vi "Scale Controls Helper.vi"(5 "rules":string, 6 "Action (Initialize)":enum16{"Initialize", "Resize", "Resize?"}(ring), 8 "error in (no error)":errorcluster, 9 "Force align? (False)":bool, 11 "vi reference":refnum<vi>) -> (0 "error out":errorcluster)   [LabVIEW 2020]
doc: "Helper VI to implement Scale Controls.vi - top level function to be called.\n\n1) Call once at GUI VI startup to initialize with action Initialize.\n2) Then call with action Resize in pane resize event to record new pane size.\n3) Then call in timeout loop with action Resize? to check if there is resize event pending and execute it. In this case the scaling rules string for Scale Controls.vi must be provided!\n\nInput parameters are static VI ref to GUI panel to be scaled in 3) the scaling rules string.\nUse 'Force align' option to force execution of scaler even if pane size not changed."
uses:
  <vilib>/Utility/miscctls.llb/LVRectTypeDef.ctl
panel:
  in  "vi list":cluster{"vi ref":refnum<vi>, "bounds":T1}[](array[cluster])
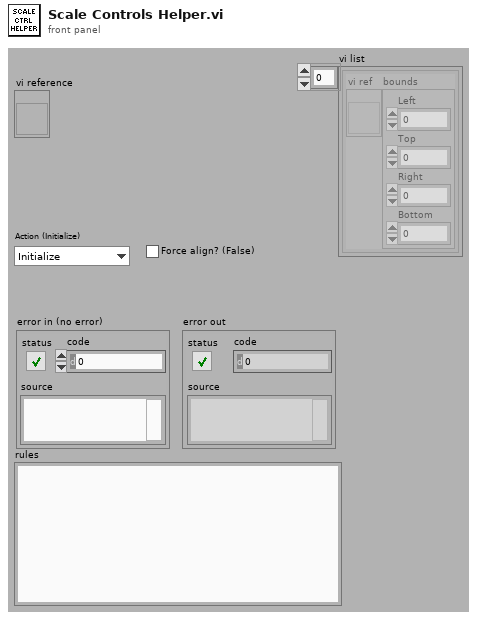
[diagram p1: front panel]
types:
  T1 = typedef "LVRectTypeDef.ctl" = cluster{"Left":i16, "Top":i16, "Right":i16, "Bottom":i16}
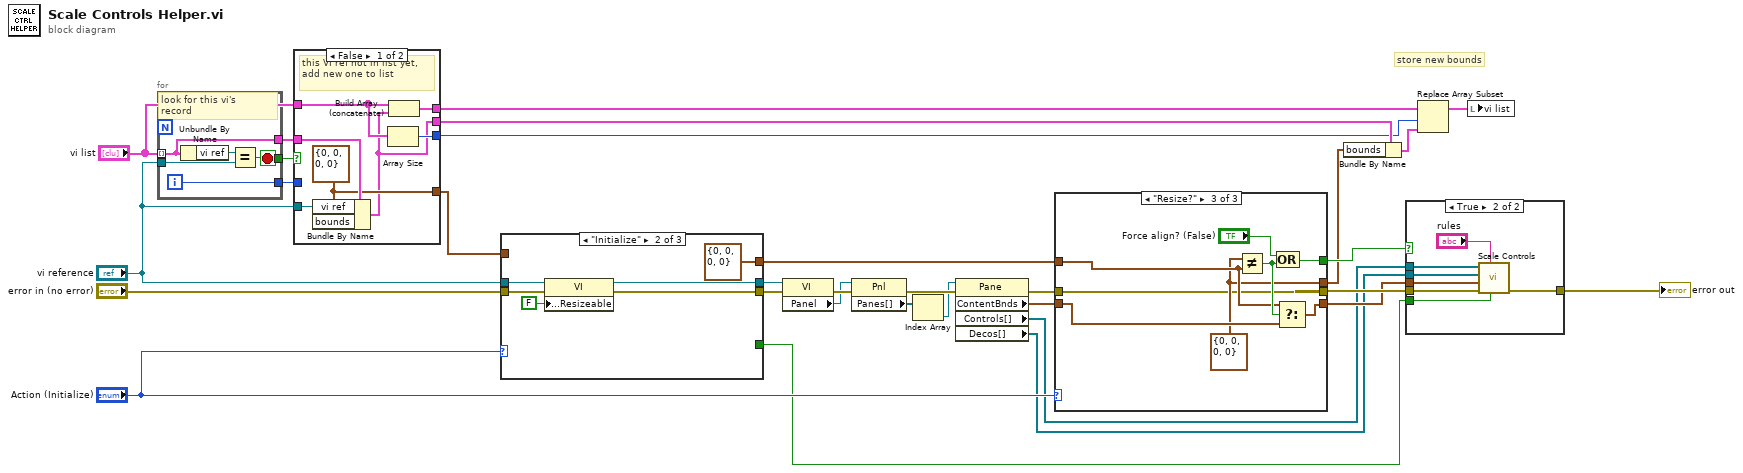
[diagram p0: block diagram]
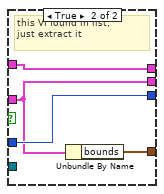
[diagram p2: hidden frame]
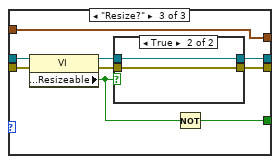
[diagram p7: hidden frame]
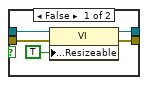
[diagram p8: hidden frame]
diagram:
  # "store new bounds"
  n1 = for {
    tunnel: "vi list" -> [w34] mode=indexing
    tunnel: "vi reference" -> [w35]
    tunnel: [w34] -> w10
    tunnel: [w33] -> w8
    tunnel: [w32] -> w12
    i -> [w33]
    stop <- w32 stop-if-true
    # "look for this vi's\nrecord"
    n2 = Unbundle By Name(w34) -> ("vi ref"=w36:refnum<vi>)
    n3 = Equal?(x=w36, y=w35) -> (x = y?=w32:bool)
  }
  n4 = case shown="False" w12 {
    tunnel: "vi list" -> [w39 w45]
    tunnel: w10 -> [w43 w44]
    tunnel: "vi reference" -> [w42 _]
    tunnel: [w41 w45] -> w7
    tunnel: [w40 w46] -> w3
    tunnel: [w38 w47] -> w4
    tunnel: w8 -> [_ w47]
    tunnel: [w37 w44] -> w6
    frame False {
      w40 = T1 {"Left"=0, "Top"=0, "Right"=0, "Bottom"=0} ("bounds")
      # "this VI ref not in list yet,\nadd new one to list"
      n5 = Bundle By Name(cluster=w43, "vi ref"=w42, "bounds"=w40) -> (w37:cluster{"vi ref":refnum<vi>, "bounds":T1})
      n6 = Array Size(array=w39) -> (size(s)=w38:i32)
      n7 = Build Array (concatenate)(w39, w37) -> (w41:cluster{"vi ref":refnum<vi>, "bounds":T1}[])
    }
    frame True {
      # "this VI found in list,\njust extract it"
      n8 = Unbundle By Name(w44) -> ("bounds"=w46:T1)
    }
  }
  n9 = case shown="\"Initialize\"" "Action (Initialize)" {
    tunnel: "error in (no error)" -> [w50 w55 w65]
    tunnel: "vi reference" -> [w49 w54 w64]
    tunnel: [w50 w51 w61] -> w29
    tunnel: [w49 w53 w60] -> w28
    tunnel: [_ _ w58] -> w15
    tunnel: w3 -> [w48 _ w57]
    tunnel: [w48 T1 {"Left"=0, "Top"=0, "Right"=0, "Bottom"=0} ("Value") w57] -> w20
    frame Default {
    }
    frame "Initialize" {
      n10 = property class="VI"(reference=w54, error in=w55, "Front Panel.Resizeable"=FALSE ("Front Panel Window:Resizable")) -> (reference out=w53:refnum<vi>, error out=w51:errorcluster)
    }
    frame "Resize?" {
      n11 = property class="VI"(reference=w64, error in=w65) -> (reference out=w62:refnum<vi>, error out=w63:errorcluster, "Front Panel.Resizeable"=w59:bool)
      n12 = case shown="True" w59 {
        tunnel: w63 -> [w70 w71]
        tunnel: w62 -> [w69 w72]
        tunnel: [w67 w71] -> w61
        tunnel: [w66 w72] -> w60
        frame False {
          n13 = property class="VI"(reference=w69, error in=w70, "Front Panel.Resizeable"=TRUE ("Front Panel Window:Resizable")) -> (reference out=w66:refnum<vi>, error out=w67:errorcluster)
        }
        frame True {
        }
      }
      n14 = Not(x=w59) -> (.not. x?=w58:bool)
    }
  }
  n15 = property class="VI"(reference=w28, error in=w29) -> (error out=w27:errorcluster, "Panel"=w26:refnum<vi>)  [unwired: 1 out]
  n16 = property class="Pnl"(reference=w26, error in=w27) -> (error out=w24:errorcluster, "Panes[]"=w25:refnum<vi>[])  [unwired: 1 out]
  n17 = Index Array(array=w25) -> (element=w23:refnum<vi>)  [unwired: 1 in]
  n18 = property class="Pane"(reference=w23, error in=w24) -> (error out=w22:errorcluster, "ContentBnds"=w21:T1, "Controls[]"=w14:refnum<vi>[], "Decos[]"=w13:refnum<vi>[])  [unwired: 1 out]
  n19 = case shown="\"Resize?\"" "Action (Initialize)" {
    tunnel: w20 -> [w73 _ w79]
    tunnel: w22 -> [w74 w76 w77]
    tunnel: w21 -> [_ w75 w81]
    tunnel: [w74 w76 w77] -> w17
    tunnel: [w73 w75 w78] -> w2
    tunnel: [_ _ w80] -> w16
    tunnel: [_ _ w84] -> w19
    frame Default {
    }
    frame "Initialize", "Resize" {
    }
    frame "Resize?" {
      w78 = T1 {"Left"=0, "Top"=0, "Right"=0, "Bottom"=0} ("Value")
      n20 = Not Equal?(x=w78, y=w79) -> (x != y?=w82:bool)
      n21 = Compound Arithmetic op=OR("Force align? (False)", w82) -> (w84:bool)
      n22 = Select(t=w79, s=w82, f=w81) -> (s? t:f=w80:T1)
    }
  }
  n23 = Bundle By Name(cluster=w6, "bounds"=w2) -> (w5:cluster{"vi ref":refnum<vi>, "bounds":T1})
  n24 = case shown="True" w19 {
    tunnel: w17 -> [w85 w92]
    tunnel: w15 -> [_ w91]
    tunnel: w16 -> [_ w90]
    tunnel: w13 -> [_ w89]
    tunnel: w14 -> [_ w88]
    tunnel: [w85 w87] -> w18
    frame False {
    }
    frame True {
      n25 = call "Scale Controls.vi"("Initialize group (false)"=w91, "rules"="rules", "error in (no error)"=w92, "pane size"=w90, "Decorations on Pane"=w89, "Controls on Pane"=w88) -> ("error out"=w87:errorcluster)  [unwired: 5 in]
    }
  }
  "error out" <- w18
  n26 = Replace Array Subset(array=w7, new element=w5, index=w4) -> (w1:cluster{"vi ref":refnum<vi>, "bounds":T1}[])
  n27 = local write "vi list"(w1) -> ()
